vi "gaussian_function.vi"(0 "X":dbl[](array[numeric]), 5 "Amplitude":dbl=1.0, 7 "sigma":dbl, 9 "mean":dbl, 11 "offset":dbl) -> (4 "Y":dbl[](array[numeric]))   [LabVIEW 2022 SP3]
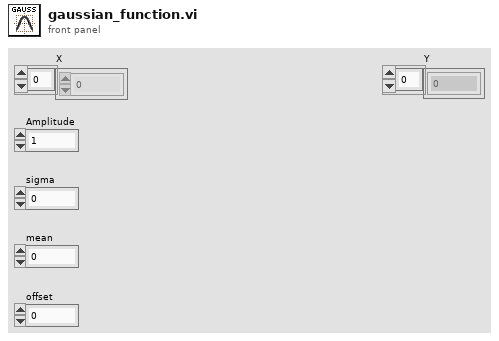
[diagram p1: front panel]
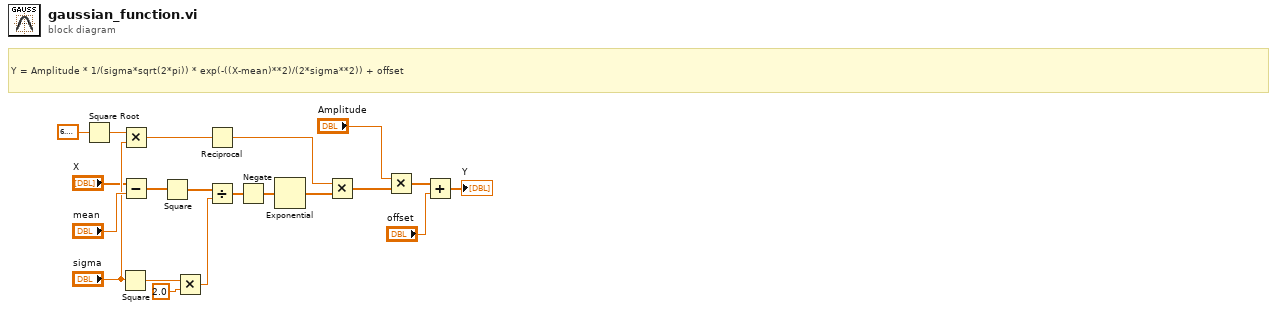
[diagram p0: block diagram]
diagram:
  # "Y = Amplitude * 1/(sigma*sqrt(2*pi)) * exp(-((X-mean)**2)/(2*sigma**2)) + offset"
  n1 = Square Root(x=6.283185307179586) -> (sqrt(x)=w19:dbl)
  n2 = Square(x="sigma") -> (x^2=w13:dbl)
  n3 = Multiply(x=w19, y="sigma") -> (x*y=w18:dbl)
  n4 = Subtract(x="X", y="mean") -> (x-y=w16:dbl[])
  n5 = Square(x=w16) -> (x^2=w15:dbl[])
  n6 = Multiply(x=w13, y=2.0) -> (x*y=w11:dbl)
  n7 = Reciprocal(x=w18) -> (1/x=w7:dbl)
  n8 = Divide(x=w15, y=w11) -> (x/y=w10:dbl[])
  n9 = Negate(x=w10) -> (-x=w9:dbl[])
  n10 = Exponential(1:w9) -> (0:w8:dbl[])
  n11 = Multiply(x=w7, y=w8) -> (x*y=w6:dbl[])
  n12 = Multiply(x="Amplitude", y=w6) -> (x*y=w4:dbl[])
  n13 = Add(x=w4, y="offset") -> (x+y=→"Y":dbl[])
